vi "Begin.vi"(8 "error in":errorcluster) -> (0 "error out":errorcluster)   [LabVIEW 2019]
doc: "Called before other user functions, this VI can be used to open I/O refnums, load in file data, and do general program initialization. Notice that the <B>error out</B> terminal is simply used for data flow. Wiring it to other structures or subVIs ensures that this VI runs first."
uses:
  <vilib>/Rock Robotics/WPI/DriverStation/WPI_DriverStationRobotMode2.ctl
  <vilib>/Rock Robotics/WPI/Joystick/WPI_JoystickDeviceEnum.ctl
  Robot Global Data.vi
  <vilib>/Rock Robotics/Network Tables/NT Write String Array.vi
  <vilib>/Rock Robotics/WPI/RobotDrive/WPI_RobotDriveOpen2MotorWithExistingMotors.vi
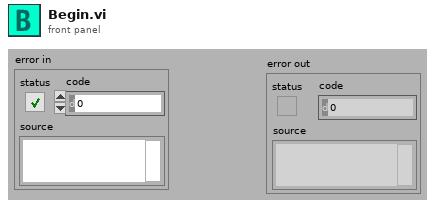
[diagram p1: front panel]
types:
  T1 = typedef "WPI_JoystickDeviceEnum.ctl" = enum16{"USB 0", "USB 1", "USB 2", "USB 3", "USB 4", "USB 5"}
  T2 = typedef "WPI_DriverStationRobotMode2.ctl" = enum16{"Autonomous Disabled", "Autonomous Enabled", "Teleop Disabled", "Teleop Enabled", "Disconnected", "Finish", "Test Disabled", "Test Enabled", "Emergency Stopped"}
  T3 = typedef "WPI_JoystickDevRef.ctl" = cluster{"Device":T1}
  T4 = typedef "WPI_MotorControlDeviceRef.ctl" = cluster{"DeviceStatus":errorcluster, "Type":T5, "PWM":cluster{"PWM Channel":T6, "DeadBand":T7}, "CAN":cluster{"Device Number":u8, "SetOutput VI Ref":variant, "GetOutput VI Ref":variant, "Enable VI Ref":variant, "Disable VI Ref":variant, "Data":variant}, "Invert":bool, "DIO PWM":cluster{"PWM \"Enable\" Channel":T6, "DIOChannel":T8, "PWM Rate":dbl}}
  T5 = typedef "WPI_MotorControlType.ctl" = enum16{"PWM", "CAN", "DIO PWM"}
  T6 = typedef "FPGA_DIOPWMChannel.ctl" = enum8{"PWM 0", "PWM 1", "PWM 2", "PWM 3", "PWM 4", "PWM 5", "PWM 6", "PWM 7", "PWM 8", "PWM 9", "PWM MXP 0", "PWM MXP 1", "PWM MXP 2", "PWM MXP 3", "PWM MXP 4", "PWM MXP 5", "PWM MXP 6", "PWM MXP 7", "PWM MXP 8", "PWM MXP 9", "Invalid"}
  T7 = typedef "WPI_PWMDeadband.ctl" = cluster{"Name":string, "maxPositivePwm":i32, "minPositivePwm":i32, "centerPwm":i32, "maxNegativePwm":i32, "minNegativePwm":i32, "angularRange":u16}
  T8 = typedef "FPGA_DIOChannel.ctl" = enum8{"DIO 0", "DIO 1", "DIO 2", "DIO 3", "DIO 4", "DIO 5", "DIO 6", "DIO 7", "DIO 8", "DIO 9", "DIO MXP 0", "DIO MXP 1", "DIO MXP 2", "DIO MXP 3", "DIO MXP 4", "DIO MXP 5", "DIO MXP 6", "DIO MXP 7", "DIO MXP 8", "DIO MXP 9", "DIO MXP 10", "DIO MXP 11", "DIO MXP 12", "DIO MXP 13", "DIO MXP 14", "DIO MXP 15", "SPI Port CS1", "SPI Port CS2", "SPI Port CS3", "SPI Port MISO", "SPI Port MOSI", "Invalid"}
  T9 = typedef "WPI_RobotDriveDevRef.ctl" = cluster{"DevStatus":errorcluster, "Motors[]":T4[], "Square Inputs":bool, "Max Output":dbl}
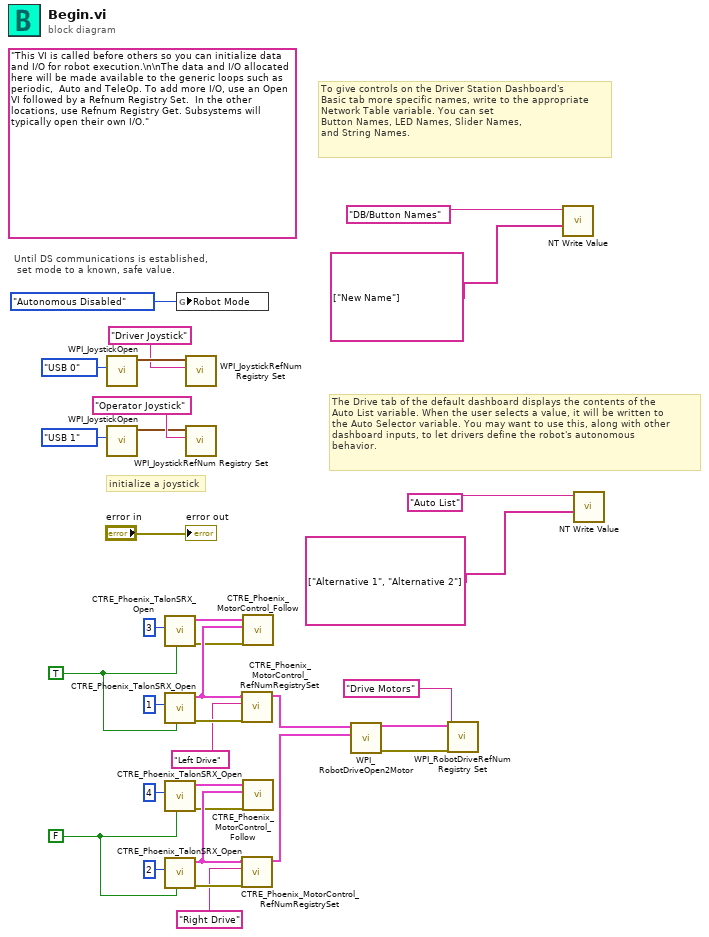
[diagram p0: block diagram]
diagram:
  w4 = FALSE ("Invert")
  w5 = TRUE ("Invert")
  (unwired) "This VI is called before others so you can initialize data and I/O for robot execution.\n\nThe data and I/O allocated here will be made available to the generic loops such as periodic,  Auto and TeleOp. To add more I/O, use an Open VI followed by a Refnum Registry Set.  In the other locations, use Refnum Registry Get. Subsystems will typically open their own I/O."
  # "The Drive tab of the default dashboard displays the contents of the\nAuto List variable. When the user selects a value, it will be written to\nthe Auto Selector variable. You may want to use this, along with other\ndashboard inputs, to let drivers define the robot's autonomous\nbehavior."
  # "To give controls on the Driver Station Dashboard's\nBasic tab more specific names, write to the appropriate\nNetwork Table variable. You can set\nButton Names, LED Names, Slider Names,\nand String Names."
  # "initialize a joystick"
  # "Until DS communications is established,\n set mode to a known, safe value."
  n1 = call <vilib>:"WPI_JoystickOpen.vi"("JoystickDevice"=WPI_JoystickDeviceEnum."USB 0") -> ("JoystickDevRef"=w2:T3)  [unwired: 10 in]
  n2 = call <vilib>:"WPI_JoystickOpen.vi"("JoystickDevice"=WPI_JoystickDeviceEnum."USB 1") -> ("JoystickDevRef"=w31:T3)  [unwired: 10 in]
  n3 = call <vilib>:"CTRE_Phoenix_TalonSRX_Open.vi"("Invert"=w5, "Device Number"=u8 3) -> ("error out"=w15:errorcluster, "CAN Talon SRX Ref"=w24:T4)  [unwired: 8 in]
  n4 = call <vilib>:"CTRE_Phoenix_TalonSRX_Open.vi"("Invert"=w5, "Device Number"=u8 1) -> ("error out"=w16:errorcluster, "CAN Talon SRX Ref"=w23:T4)  [unwired: 8 in]
  n5 = call <vilib>:"CTRE_Phoenix_TalonSRX_Open.vi"("Invert"=w4, "Device Number"=u8 4) -> ("error out"=w14:errorcluster, "CAN Talon SRX Ref"=w17:T4)  [unwired: 8 in]
  n6 = call <vilib>:"CTRE_Phoenix_TalonSRX_Open.vi"("Invert"=w4, "Device Number"=u8 2) -> ("error out"=w13:errorcluster, "CAN Talon SRX Ref"=w18:T4)  [unwired: 8 in]
  n7 = global write "Robot Global Data.vi" "Robot Mode"(WPI_DriverStationRobotMode2."Autonomous Disabled" ("Robot Mode")) -> ()
  n8 = call <vilib>:"WPI_JoystickRefNum Registry Set.vi"("refnum name"="Driver Joystick", "JoystickDevRef"=w2) -> ()  [unwired: 8 in, 2 out]
  n9 = call <vilib>:"WPI_JoystickRefNum Registry Set.vi"("refnum name"="Operator Joystick", "JoystickDevRef"=w31) -> ()  [unwired: 8 in, 2 out]
  n10 = call <vilib>:"CTRE_Phoenix_MotorControl_RefNumRegistrySet.vi"("error in (no error)"=w16, "refnum name"="Left Drive", "PhoenixMotorControlDevRef"=w23) -> ("PhoenixMotorControlDevRef"=w12:T4)  [unwired: 7 in, 1 out]
  n11 = call <vilib>:"CTRE_Phoenix_MotorControl_RefNumRegistrySet.vi"("error in (no error)"=w13, "refnum name"="Right Drive", "PhoenixMotorControlDevRef"=w18) -> ("PhoenixMotorControlDevRef"=w11:T4)  [unwired: 7 in, 1 out]
  n12 = call <vilib>:"CTRE_Phoenix_MotorControl_Follow.vi"("error in (no error)"=w15, "Master Controller to Follow"=w23, "PhoenixMotorControlDevRef"=w24) -> ()  [unwired: 7 in, 2 out]
  n13 = call <vilib>:"CTRE_Phoenix_MotorControl_Follow.vi"("error in (no error)"=w14, "Master Controller to Follow"=w18, "PhoenixMotorControlDevRef"=w17) -> ()  [unwired: 7 in, 2 out]
  n14 = call-poly <vilib>:"WPI_RobotDriveOpen2Motor.vi"("Right Motor Dev Ref"=w11, "Left Motor Dev Ref"=w12) -> ("error out"=w7:errorcluster, "RobotDriveDevRef"=w8:T9)  [unwired: 8 in]
  n15 = call <vilib>:"WPI_RobotDriveRefNum Registry Set.vi"("error in (no error)"=w7, "refnum name"="Drive Motors", "RobotDriveDevRef"=w8) -> ()  [unwired: 7 in, 2 out]
  n16 = call-poly <vilib>:"NT Write Value.vi"("String Array"=string[] ["New Name"], "Name"="DB/Button Names") -> ()  [unwired: 9 in, 1 out]
  n17 = call-poly <vilib>:"NT Write Value.vi"("String Array"=string[] ["Alternative 1", "Alternative 2"], "Name"="Auto List") -> ()  [unwired: 9 in, 1 out]
  "error out" <- "error in"
